vi "get COM name.vi"(8 "error in (no error)":errorcluster, 10 "Driver Name":string="\\Device\\VCP0") -> (0 "error out":errorcluster, 2 "COMport Name":string)   [LabVIEW 2016]
panel:
  out "values":string[](array[string])
  out "String/Binary data":string[](array[string])
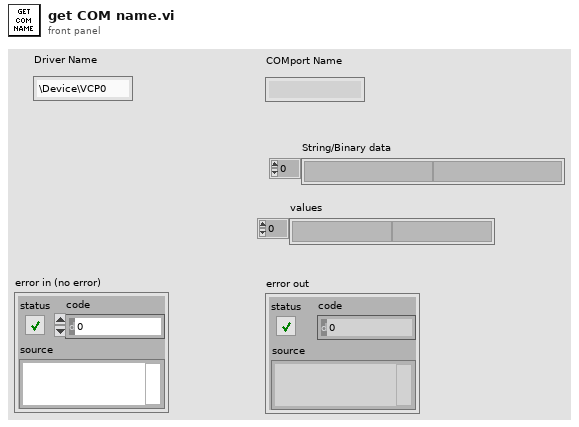
[diagram p1: front panel]
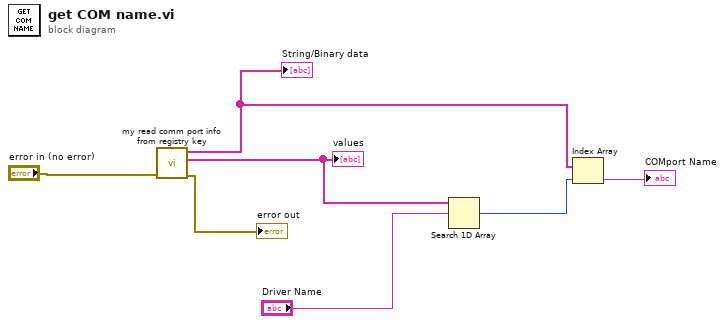
[diagram p0: block diagram]
diagram:
  n1 = call "my read comm port info from registry key.vi"("error in (no error)"="error in (no error)") -> ("error out"=→"error out":errorcluster, "values"=w4:string[], "String/Binary data"=w3:string[])  [unwired: 8 in]
  "String/Binary data" <- w3
  "values" <- w4
  n2 = Search 1D Array(1D array=w4, element="Driver Name") -> (index of element=w2:i32)  [unwired: 1 in]
  n3 = Index Array(array=w3, index=w2) -> (element=→"COMport Name":string)
